vi "I2C Write Data.vi"(5 "Address":T2 format="%02x", 6 "NoStop (F)":bool, 7 "I2C #":T1=-1, 8 "error in (no error)":errorcluster, 10 "Data":string, 11 "Session in":refnum<class "Session.lvclass">) -> (0 "error out":errorcluster, 3 "Session out":refnum<class "Session.lvclass">)   [LabVIEW 2020, in "CTI.lvlib" / "Session.lvclass"]
doc: "Writes the specified bytes out to the specified I2C bus targetted at the peripheral with the specified Address."
uses:
  Session.lvclass
  I2C Address.ctl
  I2C Number.ctl
  DeviceComms/DeviceComms.lvclass
  CTI.lvlib
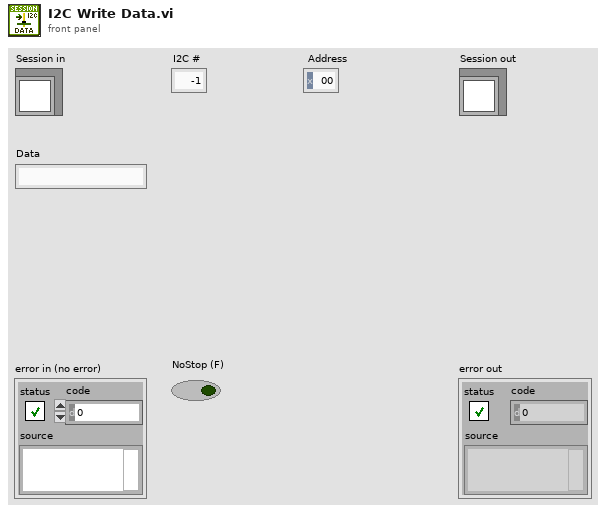
[diagram p1: front panel]
types:
  T1 = typedef "CTI.lvlib/I2C Number.ctl" = i8
  T2 = typedef "CTI.lvlib/I2C Address.ctl" = u8
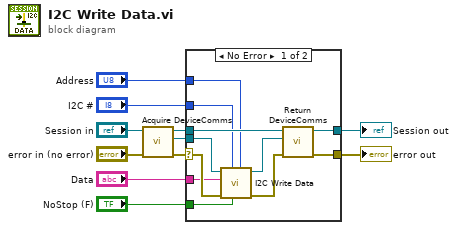
[diagram p0: block diagram]
diagram:
  n1 = call "Acquire DeviceComms.vi"("error in (no error)"="error in (no error)", "Session in"="Session in") -> ("error out"=w10:errorcluster, "DeviceComms"=w9:refnum<class "DeviceComms.lvclass">, "Session out"=w11:refnum<class "Session.lvclass">)  [unwired: 7 in]
  n2 = case shown="No Error" w10 {
    selector: w10 -> [w21 w24]
    tunnel: w11 -> [w20 w23]
    tunnel: w9 -> [w22 _]
    tunnel: [w17 w23] -> w2
    tunnel: [w16 w24] -> w1
    tunnel: "I2C #" -> [w15 _]
    tunnel: "Data" -> [w14 _]
    tunnel: "NoStop (F)" -> [w13 _]
    tunnel: "Address" -> [w12 _]
    frame No Error {
      n3 = call-dynamic "I2C Write Data.vi"("Address"=w12, "NoStop (F)"=w13, "I2C #"=w15, "error in (no error)"=w21, "Data"=w14, "DeviceComms in"=w22) -> ("error out"=w18:errorcluster, "DeviceComms out"=w19:refnum<class "DeviceComms.lvclass">)  [unwired: 4 in]
      n4 = call "Return DeviceComms.vi"("error in (no error)"=w18, "DeviceComms"=w19, "Session in"=w20) -> ("error out"=w16:errorcluster, "Session out"=w17:refnum<class "Session.lvclass">)  [unwired: 7 in]
    }
    frame Error {
    }
  }
  "error out" <- w1
  "Session out" <- w2
